vi "Write Teller.vi"(10 "Teller":refnum<class "Teller.lvclass">, 11 "Stopped Msg Input in":refnum<class "Stopped Msg Input.lvclass">) -> (3 "Stopped Msg Input out":refnum<class "Stopped Msg Input.lvclass">)   [LabVIEW 2020, in "jettl.lvlib" / "Stopped jettl Msg.lvlib" / "Stopped Msg Input.lvlib" / "Stopped Msg Input.lvclass"]
uses:
  Stopped Msg Input.lvclass
  Teller/Teller.lvclass
  Stopped Msg Input.lvclass/Stopped Msg Input.ctl
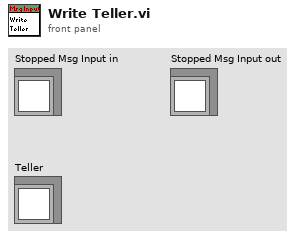
[diagram p1: front panel]
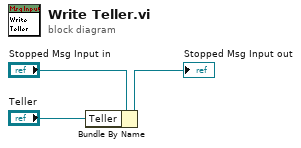
[diagram p0: block diagram]
diagram:
  n1 = Bundle By Name(cluster="Stopped Msg Input in", "Teller"="Teller") -> (→"Stopped Msg Input out":refnum<class "Stopped Msg Input.lvclass">)
